vi "SPI TxRx.vi"(8 "Error In":errorcluster, 9 "Sample Rate":dbl=10000000.0 format="%#_13p", 10 "MOSI Data":u8[](array[numeric]) format="%x", 11 "SPI Configuration In":T1={"CLK Frequency (Hz)"=250000, "CPOL"=FALSE, "CPHA"=FALSE, "CS Channel"="", "CLK Channel"="", "MOSI Channel"="", "MISO Channel"="", "Active CS"=FALSE, "Dig In Task"="", "Dig Out Task"=""} {"CLK Frequency (Hz)" format="%#.6p"}) -> (0 "Error Out":errorcluster, 1 "SPI Signals":digitalwaveform(waveform), 2 "MISO Data":u8[](array[numeric]) format="%x", 3 "SPI Configuration Out":T1={"CLK Frequency (Hz)"=250000, "CPOL"=FALSE, "CPHA"=FALSE, "CS Channel"="", "CLK Channel"="", "MOSI Channel"="", "MISO Channel"="", "Active CS"=FALSE, "Dig In Task"="", "Dig Out Task"=""} {"CLK Frequency (Hz)" format="%#.6p"})   [LabVIEW 2016, in "SPIVI.lvlib"]
uses:
  SPIVI.lvlib
  Typedefs/SPI Configuration.ctl
  <vilib>/Waveform/DWDTOps.llb/DWDT Append Digital Signals.vi
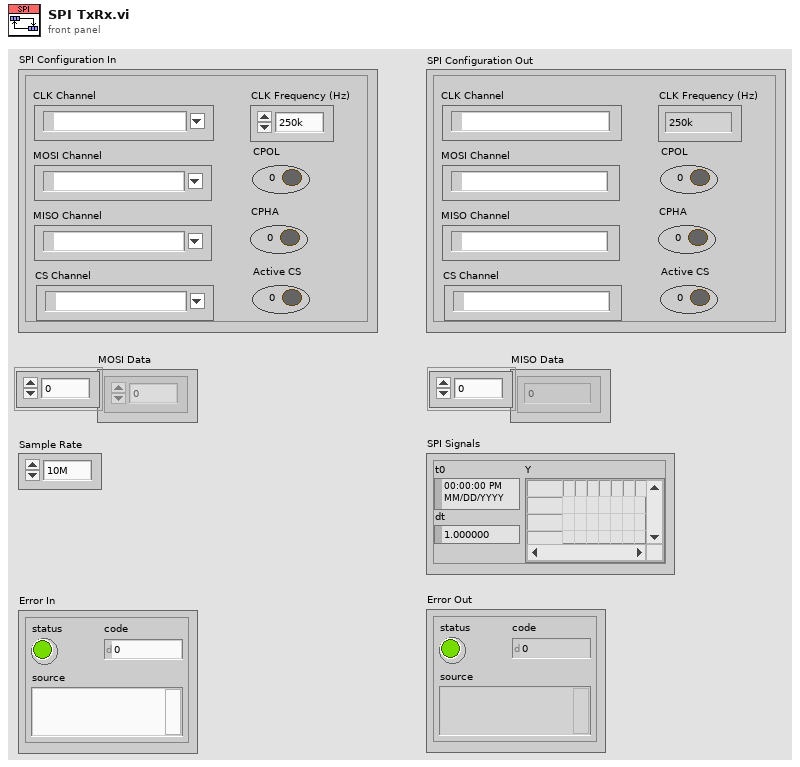
[diagram p1: front panel]
types:
  T1 = typedef "SPIVI.lvlib/SPI Configuration.ctl" = cluster{"CLK Frequency (Hz)":u32, "CPOL":bool, "CPHA":bool, "CS Channel":tag, "CLK Channel":tag, "MOSI Channel":tag, "MISO Channel":tag, "Active CS":bool, "Dig In Task":refnum<k21>, "Dig Out Task":refnum<k21>}
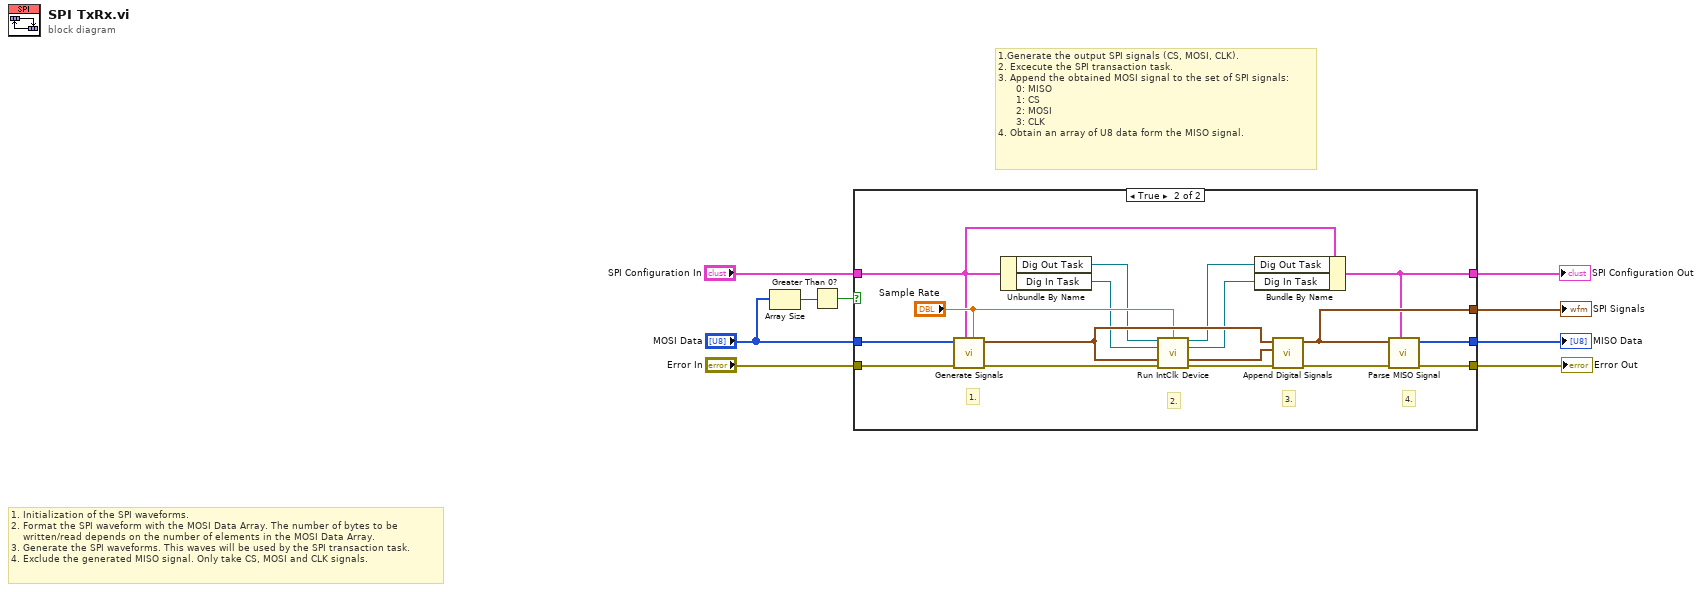
[diagram p0: block diagram]
diagram:
  # "1. Initialization of the SPI waveforms.\n2. Format the SPI waveform with the MOSI Data Array. The number of bytes to be\n    written/read depends on the number of elements in the MOSI Data Array.\n3. Generate the SPI waveforms. This waves will be used by the SPI transaction task.\n4. Exclude the generated MISO signal. Only take CS, MOSI and CLK signals."
  # "1.Generate the output SPI signals (CS, MOSI, CLK).\n2. Excecute the SPI transaction task.\n3. Append the obtained MOSI signal to the set of SPI signals:\n      0: MISO\n      1: CS\n      2: MOSI\n      3: CLK\n4. Obtain an array of U8 data form the MISO signal."
  n1 = Array Size(array="MOSI Data") -> (size(s)=w1:i32)
  n2 = Greater Than 0?(x=w1) -> (x > 0?=w2:bool)
  n3 = case shown="True" w2 {
    tunnel: "Error In" -> [w10 w26]
    tunnel: [w10 w22] -> w8
    tunnel: [_ w21] -> w7
    tunnel: [_ w20] -> w6
    tunnel: "MOSI Data" -> [_ w18]
    tunnel: "SPI Configuration In" -> [w11 w13]
    tunnel: [w11 w12] -> w4
    frame False {
    }
    frame True {
      # "4."
      # "1."
      # "3."
      # "2."
      n4 = call "Generate Signals.vi"("Sample Rate"="Sample Rate", "SPI Configuration"=w13, "Error In"=w26, "MOSI Data"=w18) -> ("Error Out"=w25:errorcluster, "Signals"=w24:digitalwaveform)  [unwired: 6 in]
      n5 = Unbundle By Name(w13) -> ("Dig Out Task"=w17:refnum<k21>, "Dig In Task"=w16:refnum<k21>)
      n6 = call "Run IntClk Device.vi"("Dig out task"=w17, "Oversample clock rate"="Sample Rate", "Dig in task"=w16, "Digital waveform"=w24, "error in (no error)"=w25) -> ("Dig out task out"=w15:refnum<k21>, "Dig in task out"=w14:refnum<k21>, "Input ch data"=w28:digitalwaveform, "error out"=w27:errorcluster)  [unwired: 7 in]
      n7 = Bundle By Name(cluster=w13, "Dig Out Task"=w15, "Dig In Task"=w14) -> (w12:T1)
      n8 = call-poly <vilib>:"Append Digital Signals.vi"("error in (no error)"=w27, "digital waveform (low bits)"=w28, "digital waveform (high bits)"=w24) -> ("error out"=w23:errorcluster, "digital waveform out"=w20:digitalwaveform)  [unwired: 7 in]
      n9 = call "Parse MISO Signal.vi"("SPI Configuration"=w12, "Error In"=w23, "SPI Signals"=w20) -> ("Error Out"=w22:errorcluster, "MISO Data"=w21:u8[])  [unwired: 7 in]
    }
  }
  "SPI Signals" <- w6
  "Error Out" <- w8
  "MISO Data" <- w7
  "SPI Configuration Out" <- w4
